vi "Read Obs.vi"(8 "error in (no error)":errorcluster, 11 "Obs Based Step in":refnum<class "Obs Based Step.lvclass">) -> (0 "error out":errorcluster, 2 "Obs":u16, 3 "Obs Based Step out":refnum<class "Obs Based Step.lvclass">)   [LabVIEW 2015, in "Obs Based Step.lvclass"]
uses:
  Obs Based Step.lvclass
  Obs Based Step.lvclass/Obs Based Step.ctl
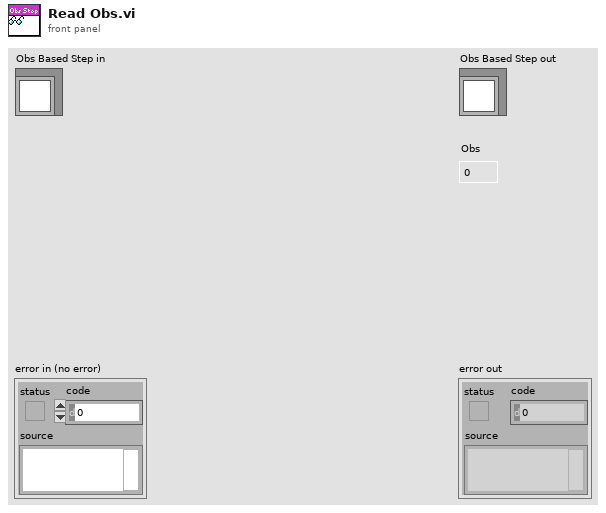
[diagram p1: front panel]
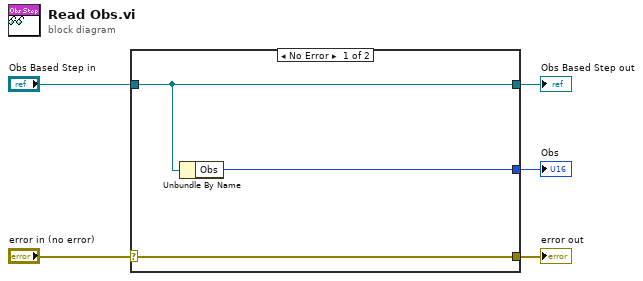
[diagram p0: block diagram]
diagram:
  n1 = case shown="No Error" "error in (no error)" {
    selector: "error in (no error)" -> [w8 w9]
    tunnel: [w8 w9] -> w4
    tunnel: [w7 w10] -> w2
    tunnel: "Obs Based Step in" -> [w7 w10]
    tunnel: [w6 _] -> w1
    frame No Error {
      n2 = Unbundle By Name(w7) -> ("Obs"=w6:u16)
    }
    frame Error {
    }
  }
  "error out" <- w4
  "Obs Based Step out" <- w2
  "Obs" <- w1
